vi "dane z WmF.vi"(8 "error in (no error)":errorcluster, 11 "Przebiegi in":T1) -> (0 "error out":errorcluster, 2 "przebiegi":waveform(dbl)[](array[waveform]), 3 "Nazwy":string[](array[string]), 4 "Kanaly":string, 5 "rozm":i32)   [LabVIEW 2013]
uses:
  Kontrolki/Przetwarzanie/Kanaly.ctl
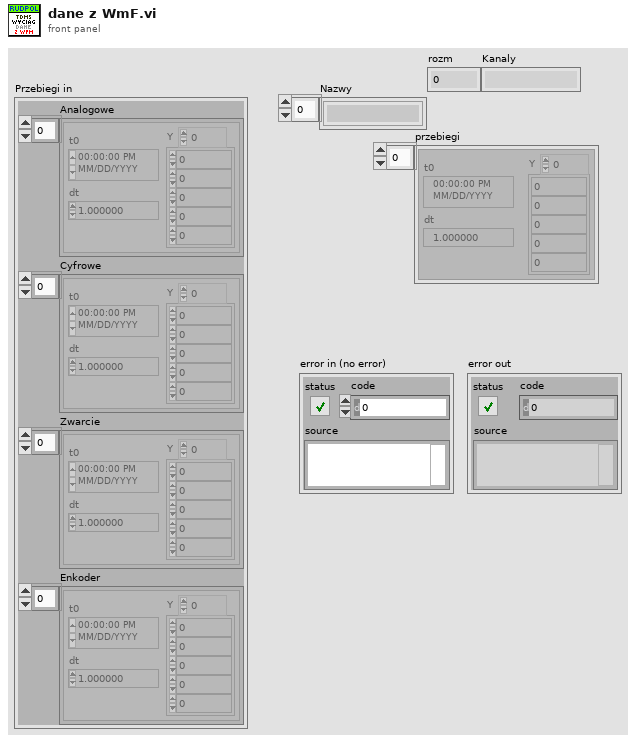
[diagram p1: front panel]
types:
  T1 = typedef "Kanaly.ctl" = cluster{"Analogowe":waveform(dbl)[], "Cyfrowe":waveform(dbl)[], "Zwarcie":waveform(dbl)[], "Enkoder":waveform(dbl)[]}
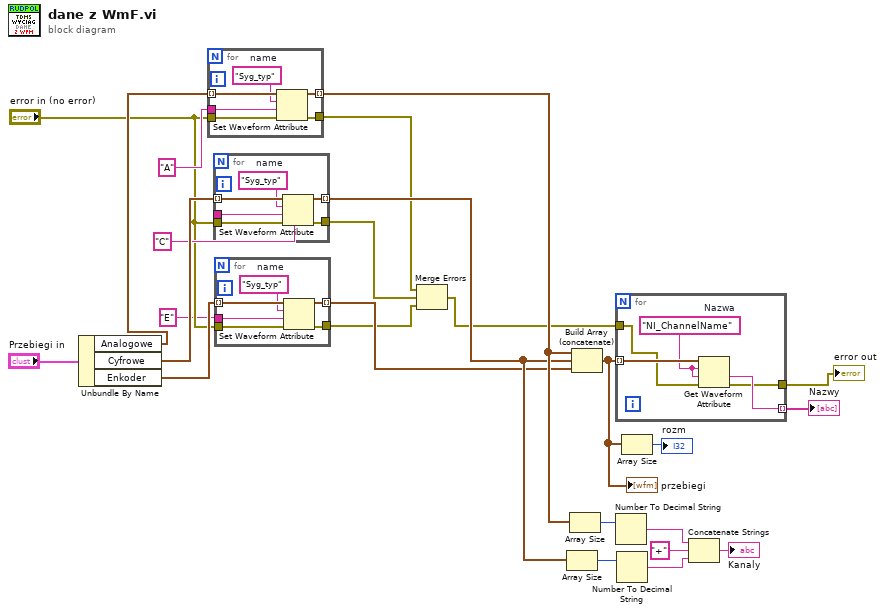
[diagram p0: block diagram]
diagram:
  n1 = Unbundle By Name("Przebiegi in") -> ("Analogowe"=w15:waveform(dbl)[], "Cyfrowe"=w12:waveform(dbl)[], "Enkoder"=w9:waveform(dbl)[])
  n2 = for {
    tunnel: w15 -> [w31] mode=indexing
    tunnel: "error in (no error)" -> [w29]
    tunnel: [w28] -> w14 mode=indexing
    tunnel: [w27] -> w5
    tunnel: "A" ("Nazwa") -> [w26]
    w30 = "Syg_typ"  # name
    n3 = Set Waveform Attribute(4:w29, 5:w26, 6:w30, 7:w31) -> (0:w27:errorcluster, 3:w28:waveform(dbl))  [unwired: 1 out]
  }
  n4 = for {
    tunnel: w12 -> [w37] mode=indexing
    tunnel: "error in (no error)" -> [w35]
    tunnel: [w34] -> w10 mode=indexing
    tunnel: [w33] -> w4
    tunnel: "C" ("Nazwa") -> [w32]
    w36 = "Syg_typ"  # name
    n5 = Set Waveform Attribute(4:w35, 5:w32, 6:w36, 7:w37) -> (0:w33:errorcluster, 3:w34:waveform(dbl))  [unwired: 1 out]
  }
  n6 = for {
    tunnel: w9 -> [w43] mode=indexing
    tunnel: "error in (no error)" -> [w41]
    tunnel: [w40] -> w8 mode=indexing
    tunnel: [w39] -> w3
    tunnel: "E" ("Nazwa") -> [w38]
    w42 = "Syg_typ"  # name
    n7 = Set Waveform Attribute(4:w41, 5:w38, 6:w42, 7:w43) -> (0:w39:errorcluster, 3:w40:waveform(dbl))  [unwired: 1 out]
  }
  n8 = Merge Errors(w5, w4, w3) -> (w2:errorcluster)
  n9 = Array Size(array=w10) -> (size(s)=w20:i32)
  n10 = Array Size(array=w14) -> (size(s)=w21:i32)
  n11 = Build Array (concatenate)(w14, w10, w8) -> (w23:waveform(dbl)[])
  "przebiegi" <- w23
  n12 = for {
    tunnel: w23 -> [w48] mode=indexing
    tunnel: [w46] -> w25 mode=indexing
    tunnel: w2 -> [w45]
    tunnel: [w44] -> w1
    w47 = "NI_ChannelName"  # Nazwa
    n13 = Get Waveform Attribute(4:w45, 5:w47, 6:w47, 7:w48) -> (0:w44:errorcluster, 1:w46:string)  [unwired: 2 out]
  }
  "Nazwy" <- w25
  "error out" <- w1
  n14 = Number To Decimal String(number=w21) -> (decimal integer string=w19:string)  [unwired: 1 in]
  n15 = Number To Decimal String(number=w20) -> (decimal integer string=w18:string)  [unwired: 1 in]
  n16 = Array Size(array=w23) -> (size(s)=→"rozm":i32)
  n17 = Concatenate Strings(w19, "+" ("string"), w18) -> (→"Kanaly":string)
